vi "Swap Elements Demo.vi"(11 "error in":errorcluster) -> (4 "swapped doubles":dbl[](array[numeric]), 6 "swapped strings":string[](array[string]), 15 "error out":errorcluster)   [LabVIEW 2026]
doc: "Calls Swap Elements.vim twice with two different element types, to show one malleable VI serving both."
uses:
  da08b032-a256-4283-8e39-bf10875cc60f.vi
  7c900593-026b-4dd8-a578-03710ea4ba66.vi
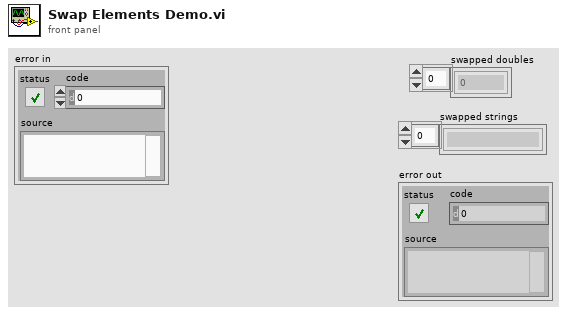
[diagram p1: front panel]
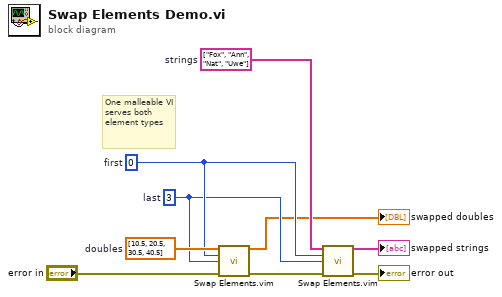
[diagram p0: block diagram]
diagram:
  w5 = 3  # last
  w6 = 0  # first
  w7 = string[] ["Fox", "Ann", "Nat", "Uwe"]  # strings
  w9 = dbl[] [10.5, 20.5, 30.5, 40.5]  # doubles
  # "One malleable VI serves both element types"
  n1 = call "Swap Elements.vim"("array in"=w9, "index A"=w6, "index B"=w5, "error in"="error in") -> ("array out"=→"swapped doubles":dbl[], "error out"=w4:errorcluster)  [unwired: 10 in]
  n2 = call "Swap Elements.vim"("array in"=w7, "index A"=w6, "index B"=w5, "error in"=w4) -> ("array out"=→"swapped strings":string[], "error out"=→"error out":errorcluster)  [unwired: 10 in]
